vi "InitAIO.vi"(8 "error in (no error)":errorcluster, 9 "CardID":u32, 10 "CardName":string, 11 "AIO in":refnum<class "AIO.lvclass">) -> (0 "error out":errorcluster, 3 "AIO out":refnum<class "AIO.lvclass">)   [LabVIEW 2024, in "AIO Actor.lvlib" / "AIO.lvclass"]
uses:
  AIO.lvclass
  AO Type.ctl
  AIO.lvclass/AIO.ctl
panel:
  in  "AoValue":T2
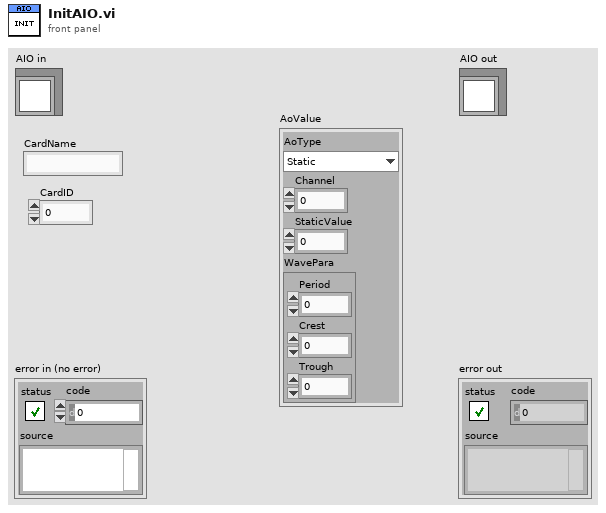
[diagram p1: front panel]
types:
  T1 = typedef "AO Type.ctl" = enum16{"Static", "Streaming", "StopStreaming"}
  T2 = cluster{"AoType":T1, "Channel":u8, "StaticValue":dbl, "WavePara":cluster{"Crest":dbl, "Trough":dbl, "Period":dbl}}
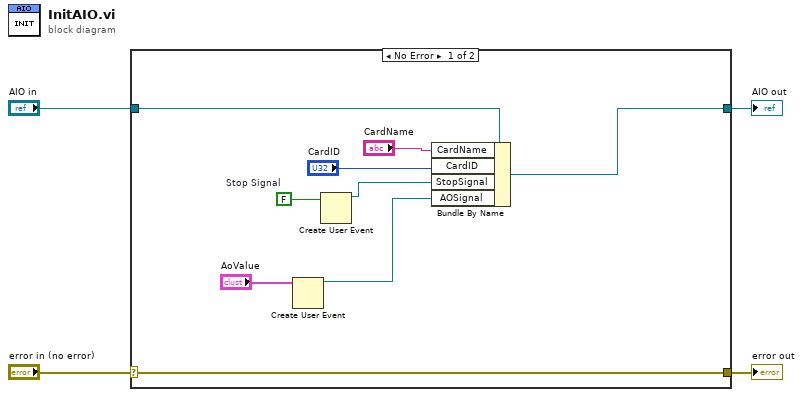
[diagram p0: block diagram]
diagram:
  n1 = case shown="No Error" "error in (no error)" {
    selector: "error in (no error)" -> [w13 w15]
    tunnel: [w13 w15] -> w3
    tunnel: [w5 w14] -> w1
    tunnel: "AIO in" -> [w6 w14]
    frame No Error {
      w9 = FALSE  # Stop Signal
      n2 = Create User Event(user event datatype="AoValue") -> (user event=w7:refnum<user-event>)  [unwired: 1 in, 1 out]
      n3 = Create User Event(user event datatype=w9) -> (user event=w8:refnum<user-event>)  [unwired: 1 in, 1 out]
      n4 = Bundle By Name(cluster=w6, "CardName"="CardName", "CardID"="CardID", "StopSignal"=w8, "AOSignal"=w7) -> (w5:refnum<class "AIO.lvclass">)
    }
    frame Error {
    }
  }
  "error out" <- w3
  "AIO out" <- w1
